vi "MouseDown Response.vi"(4 "PlatMods":T1, 6 "Mods":cluster{"Double Click":bool, "Menu Key":bool}, 8 "error in (no error)":errorcluster, 9 "Button":u16, 10 "Coords":T2, 11 "Editor Handler in":refnum<class "Image Editor Handler.lvclass">) -> (0 "error out":errorcluster, 3 "Editor Handler out":refnum<class "Image Editor Handler.lvclass">)   [LabVIEW 2015, in "LV Image Editor Framework.lvlib" / "Image Editor Handler.lvclass"]
uses:
  Image Editor Handler.lvclass
  <vilib>/Utility/miscctls.llb/LVPoint32TypeDef.ctl
  Image Editor Handler.lvclass/Image Editor Handler.ctl
  Forms/Shape/Shape.lvclass
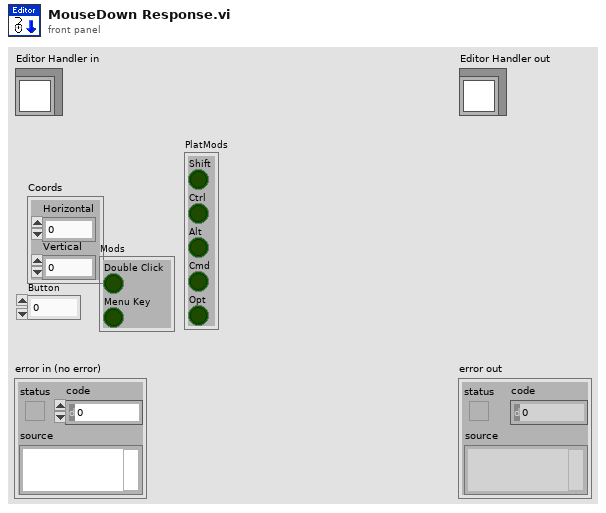
[diagram p1: front panel]
types:
  T1 = cluster{"Shift":bool, "Ctrl":bool, "Alt":bool, "Cmd":bool, "Opt":bool}
  T2 = typedef "LVPoint32TypeDef.ctl" = cluster{"Horizontal":i32, "Vertical":i32}
  T3 = typedef "LVPositionTypeDef.ctl" = cluster{"Left":i32, "Top":i32}
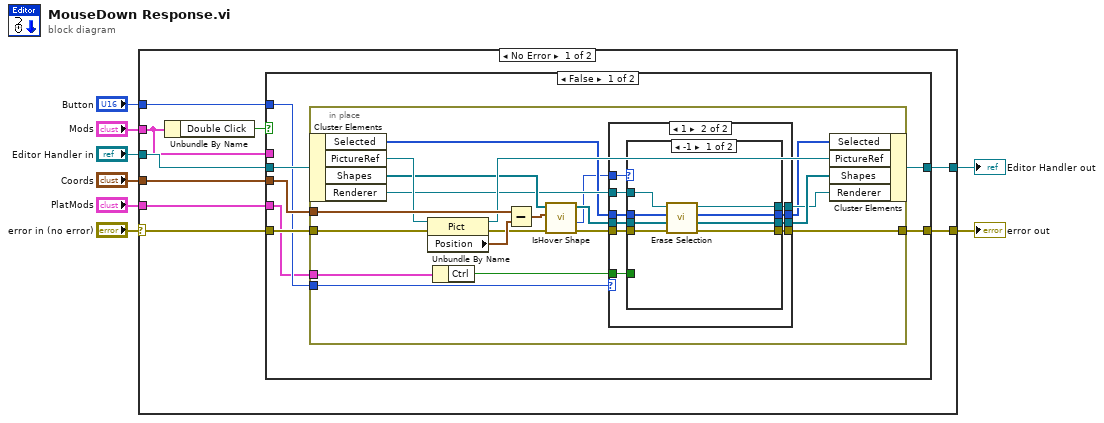
[diagram p0: block diagram]
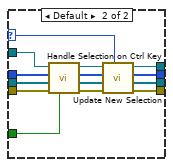
[diagram p3: hidden frame]
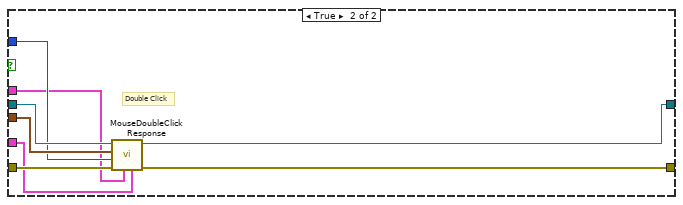
[diagram p4: hidden frame]
diagram:
  n1 = case shown="No Error" "error in (no error)" {
    selector: "error in (no error)" -> [w17 w90]
    tunnel: [w13 w90] -> w7
    tunnel: [w12 w89] -> w5
    tunnel: "Editor Handler in" -> [w15 w89]
    tunnel: "Coords" -> [w16 _]
    tunnel: "Button" -> [w14 _]
    tunnel: "PlatMods" -> [w11 _]
    tunnel: "Mods" -> [w9 _]
    frame No Error {
      n2 = Unbundle By Name(w9) -> ("Double Click"=w10:bool)
      n3 = case shown="False" w10 {
        tunnel: w17 -> [w24 w85]
        tunnel: w16 -> [w23 w87]
        tunnel: w15 -> [w22 w88]
        tunnel: w14 -> [w21 w86]
        tunnel: [w20 w84] -> w13
        tunnel: [w19 w83] -> w12
        tunnel: w11 -> [w18 w81]
        tunnel: w9 -> [_ w82]
        frame False {
          n4 = in-place {
            in-place-border: w24 -> [w44]
            in-place-border: w23 -> [w43]
            in-place-border: w21 -> [w25]
            in-place-border: [w34] -> w20
            in-place-border: w18 -> [w27]
            n5 = in-place-cluster #1(w22) -> ("Selected"=w30:i16[], "PictureRef"=w40:refnum<vi>, "Shapes"=w38:refnum<data-value>[], "Renderer"=w32:refnum<class "Image.lvclass">)
            n6 = property class="Pict"(reference=w40, error in=w44) -> (reference out=w39:refnum<vi>, error out=w37:errorcluster, "Position"=w42:T3)
            n7 = Unbundle By Name(w27) -> ("Ctrl"=w26:bool)
            n8 = Subtract(x=w43, y=w42) -> (x-y=w41:T2)
            n9 = call "IsHover Shape.vi"("error in (no error)"=w37, "Coords"=w41, "Shape in"=w38) -> ("error out"=w33:errorcluster, "Node ID"=w28:i32, "Shape out"=w36:refnum<data-value>[])  [unwired: 5 in, 1 out]
            n10 = case shown="1" w25 {
              tunnel: w36 -> [w46 w58]
              tunnel: [w46 w57] -> w35
              tunnel: [w45 w56] -> w34
              tunnel: w33 -> [w45 w55]
              tunnel: w32 -> [w47 w54]
              tunnel: [w47 w53] -> w31
              tunnel: w30 -> [w48 w52]
              tunnel: [w48 w51] -> w29
              tunnel: w28 -> [_ w50]
              tunnel: w26 -> [_ w49]
              frame Default {
                # "Other than left click"
              }
              frame 1 {
                n11 = case shown="-1" w50 {
                  selector: w50 -> [_ w69]
                  tunnel: w58 -> [w66 w74]
                  tunnel: [w64 w80] -> w57
                  tunnel: [w59 w79] -> w56
                  tunnel: w55 -> [w60 w70]
                  tunnel: w54 -> [w65 w73]
                  tunnel: [w63 w78] -> w53
                  tunnel: w52 -> [w62 w75]
                  tunnel: [w61 w77] -> w51
                  tunnel: w49 -> [_ w76]
                  frame -1 {
                    n12 = call "Erase Selection.vi"("error in (no error)"=w60, "Shape in"=w66, "Selected in"=w62, "Image in"=w65) -> ("error out"=w59:errorcluster, "Shape out"=w64:refnum<data-value>[], "Selected out"=w61:i16[], "Image out"=w63:refnum<class "Image.lvclass">)  [unwired: 4 in]
                  }
                  frame Default {
                    n13 = call "Handle Selection on Ctrl Key.vi"("Ctrl"=w76, "error in (no error)"=w70, "Shape in"=w74, "Selected in"=w75, "Image in"=w73) -> ("error out"=w71:errorcluster, "Shape out"=w67:refnum<data-value>[], "Selected out"=w68:i16[], "Image out"=w72:refnum<class "Image.lvclass">)  [unwired: 3 in]
                    n14 = call "Update New Selection.vi"("Node ID"=w69, "error in (no error)"=w71, "Shape in"=w67, "Selected in"=w68, "Image in"=w72) -> ("error out"=w79:errorcluster, "Shape out 2"=w80:refnum<data-value>[], "Selected out 2"=w77:i32[], "Image out"=w78:refnum<class "Image.lvclass">)  [unwired: 3 in]
                  }
                }
              }
            }
            n15 = in-place-cluster #1("Selected"=w29, "PictureRef"=w39, "Shapes"=w35, "Renderer"=w31) -> (w19:refnum<class "Image Editor Handler.lvclass">)
          }
        }
        frame True {
          # "Double Click"
          n16 = call-dynamic "MouseDoubleClick Response.vi"("PlatMods"=w81, "Mods"=w82, "error in (no error)"=w85, "Button"=w86, "Coords"=w87, "Editor Handler in"=w88) -> ("error out"=w84:errorcluster, "Editor Handler out"=w83:refnum<class "Image Editor Handler.lvclass">)  [unwired: 4 in]
        }
      }
    }
    frame Error {
    }
  }
  "error out" <- w7
  "Editor Handler out" <- w5
